vi "daq_run.vi"() -> ()   [LabVIEW 2011]
uses:
  <vilib>/DAQmx/read.llb/DAQmx Read (Analog 1D Wfm NChan NSamp).vi
  <vilib>/DAQmx/miscellaneous.llb/DAQmx Fill In Error Info.vi
  C:/Program Files (x86)/National Instruments/LabVIEW 2011/resource/objmgr/daqmx.rc
  <vilib>/Analysis/NI_AALBase.lvlib
panel:
  in  "Tab Control":T1(tab)=enum."Start DAQ and Nulling"
  in  "X-factor":dbl[](array[numeric])=[22.48, 0.9]
  in  "Strain Offset Nulling":bool
  in  "Shunting Calibration?":bool caption="Shunting Calibration? (DO after nulling)"
  in  "Offset reading":bool
  out "Null_offset":dbl[](array[numeric])=[0.01475870289296967, -9.76222778184623e-05]
  out "Gain adjust":dbl[](array[numeric])
  in  "Sample to read each time":i32=20
  in  "Measure actual excitation?":bool
  in  "Shunt Resistance":dbl=100000.0 format="%0.2f"
  in  "Shunt Location":enum32{"R1", "R2", "R3", "R4"}(ring)=enum."R3"
  out "VOLTAGE":dbl[][](graph)=[[0.3317756410339582, -8.786005003661606e-05]] caption="Voltage based transducer Reading"
  out "Strain Value":dbl[][](graph) caption="Strain gauge readings"
  out "Voltage":dbl[](array[numeric])=[0.3317756410339582, -8.786005003661606e-05]
  out "Strain":dbl[](array[numeric])
  out "Available data points each channel \n(too big will cause overflow problem)":u32
  in  "Record\nfull data to file":bool
  out "Offset indicator":bool
  out "Available data points each channel \n(too big will cause overflow problem) 2":u32
  in  "names in 2":string[](array[string])
  in  "gain":dbl format="%0.2f"
  in  "Boolean":bool
  in  "names in":string[](array[string])
  in  "index":i32
  in  "Path":path
  # "USER's INSTRUCTIONS\n\n1. This Version of of DAQ was developed based on the following hardware combination. Use any of the hardware outside of the following list need further verification \n--- PCI-MIO-16E-4\n--- NI-SCXI-1000/1001\n--- NI-SCXI-1520\n--- NI-SCXI-1314\n\n2. General Steps to use this DAQ software\nStep 1: Click to run the main program (DAQ has not been started yet)\nStep 2: Go over the 'Voltage Channel Initialize' and 'Strain Channel initialize' tab to make  \n             the measurement settings.  click the 'Do parsameter initialize' at least once to set \n             total channels need for voltage and strain, and then change to the right setting.\nStep 3: After all settings, go 'Start DAQ and Nulling' tab and select the sampling rate. After \n             that switch on the 'Start DAQ' button (Will show as green). It is only valid once,if \n             someting goes wrong, abort the execution and run the program again. You can \n             directly approach to Step 3 if all settings in step 2 are correct.\nStep 4: If there is at least one strain gauge channel, hit 'strain offset nulling'  and wait until \n             the gren light turned off. Then shnut calibrate the gauges if need. Finally, turn on \n              'offset reading' to zero the voltage based results. (The ligh will and should be \n             lighted during the following steps.\nStep 5:  Go to tab 'Data monitoring and recording' to see the real time collected data, The \n              voltaged based transducer readings and the strain gauge readings are shown in  \n              separate plots. The Volatge based transducer show the factored value in specific \n              units and the strain shown in microstrain.  \nStep 6: If the data is correctly read. Do the following to initialize the testing:\n             1) Zero the loading machine transducer (UTM,MTS)\n             2) repeat Step 4,5 to rezero all readings in DAQ.\n             3) Click 'Record full data to file' button under 'Data Monitoring and recording' tab\n             4) Run the testing procedure built in UTM or MTS.\nStep 7: Use 'Custom_plot' tab to plot any x versus y plot during the test. \n             USe reset graph to replot, ( the replot will NOT affect the data recording)\nStep 8: turn off the program using 'Start DAQ' button. The data recording to file will switch \n              off simutaneously.\nStep 9: Rename the recorded file, the original name will be this vi file name with 'lvm' \n             extension, can be open with MS.excel\n3. hardware settings\n     Correct Hardware connections are impotant to successul DAQ work. And the setting need to be corresponding to the software settings. The following are common settings:\n\n            1) Pure Voltage (TUM,MTS load and disp export)  :  Half bridge with excitation lead \n                                      unwire)\n            2) Potential meters :  Half bridge with exciation lead wired\n            \n            3) Strain gauge: (Quarter bridge type II is the most commonly used)\n                  See cover of SCXI-1314 for lead connection type for different gauges\nIt is always a good practice to open cover and check the wiring if not sure about that\n\nCOPY this file with 'myshunt.dll' if want to work at other directory\n\n\n4 For more information, check the documents."
  # "Version 2010.5.1\nWrote and compiled by Jun\nemail:xiajun19800812@hotmail.com"
  # "reading scale"
  # "Predefined y=x custom scale"
  # "user factors"
  # "Name and pyhsical channel"
  # "Exciations"
  # "Strain Gauge information"
  # "Reading range"
  # "Channel name and physical address"
  # "bridge settings"
  # "Sampling Frequency, recorded data time spacing is [1/(n2/n1)] second"
  # "Start DAQ"
  # "n1, the number of data to be averaged"
  # "n2, The number collect by DAQ per second"
  # "Strain Channel nulling and shunt calibration"
  # "All Channel numerical offset to zero"
  # "Shunt Calibration information"
  # "Record to file in progress\nWarning:Existing file will be overwrite, change the name below"
  # "Numerical offset in progress"
  # "Peak Valley Detection"
  # "Step 1: Set initial cycle number"
  # "Step 2: Setup cycle detecting alogrithm"
  # "Data Recording"
  # "Step 3: Setup data file recording"
  # "Recording every N cycles for M continuous cycles\nRecord First I cycles completely"
  # "Step 4: Specimen name and start fatigue DAQ"
  # "Remember to create this folder first"
  # "Fatigue recorded file loader"
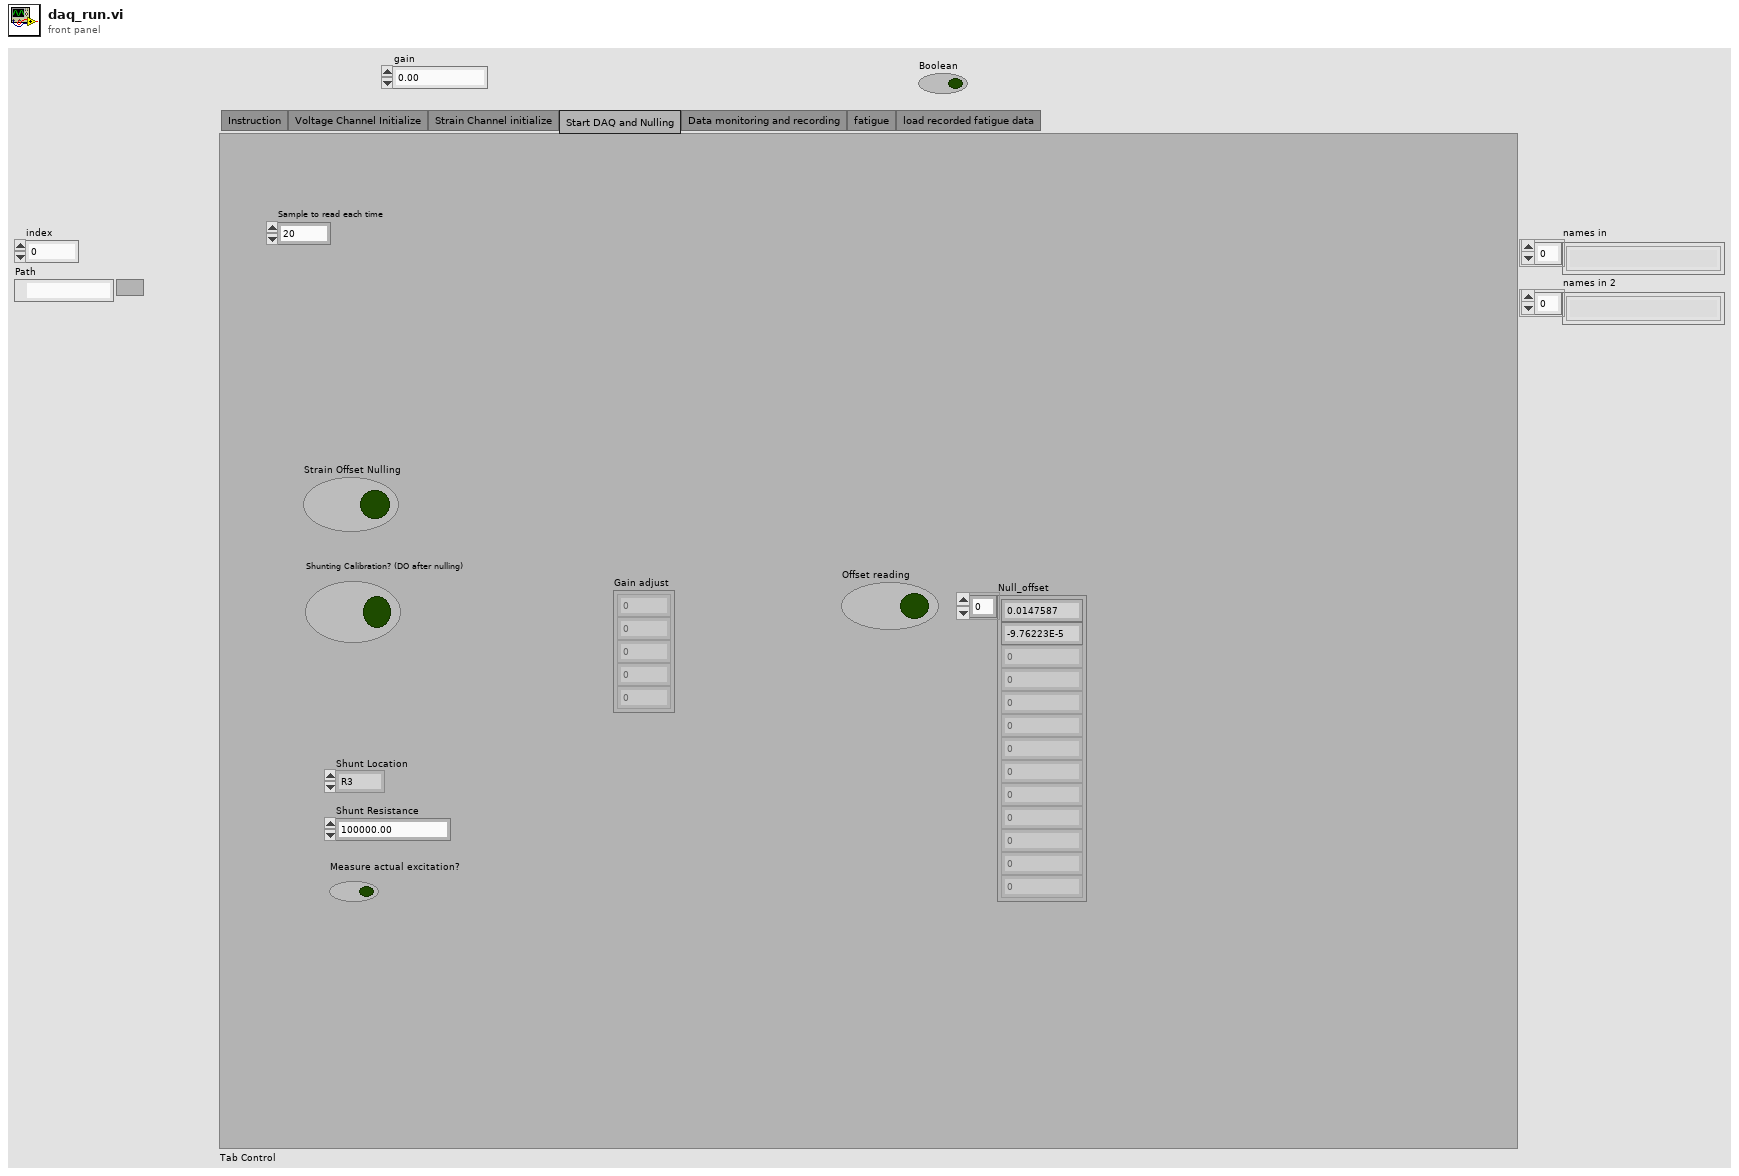
[diagram p1: front panel]
types:
  T1 = enum32{"Instruction", "Voltage Channel Initialize", "Strain Channel initialize", "Start DAQ and Nulling", "Data monitoring and recording", "fatigue", "load recorded fatigue data"}
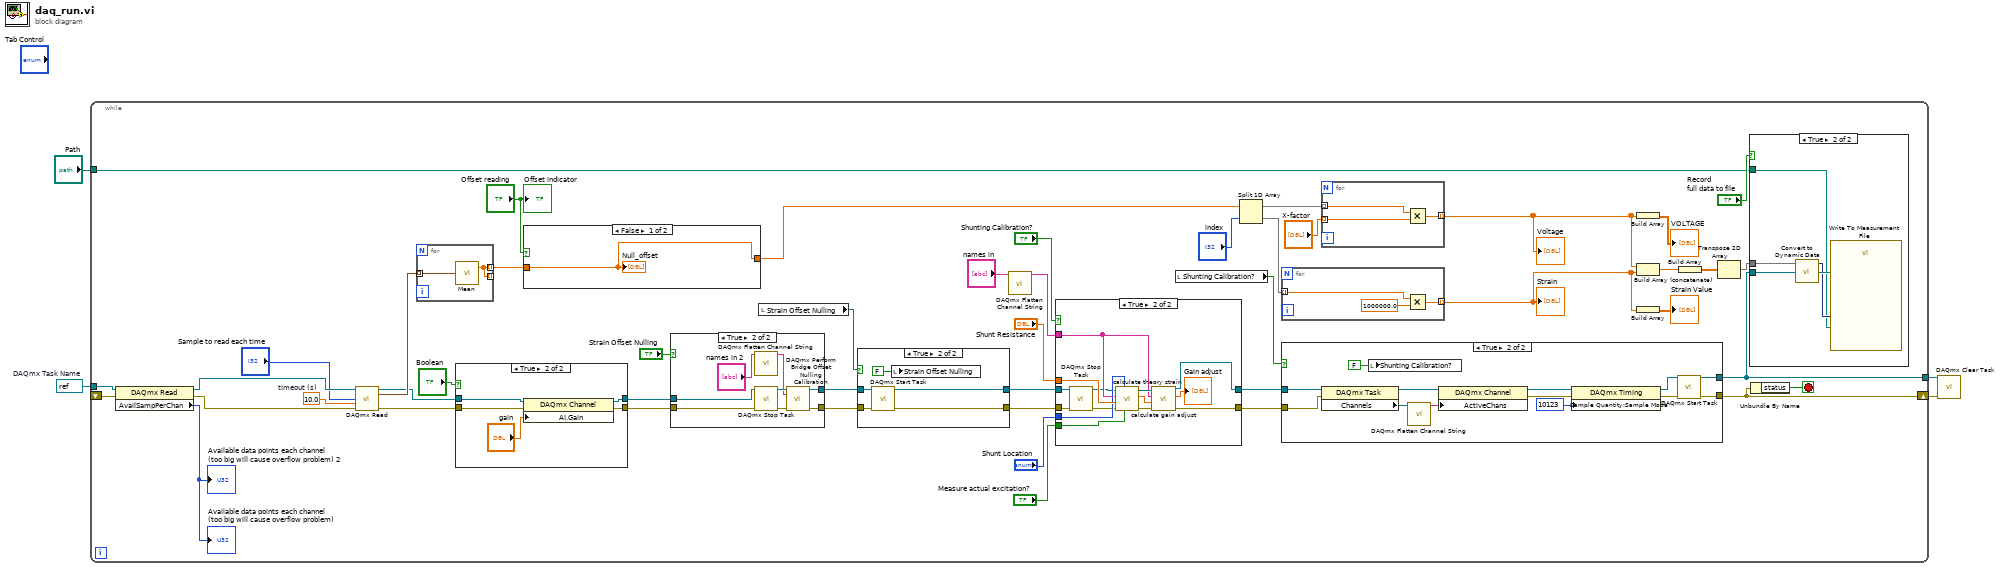
[diagram p0: block diagram]
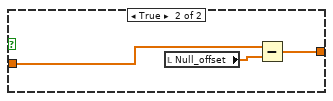
[diagram p3: hidden frame]
diagram:
  w2 = refnum<k21> refnum  # DAQmx Task Name
  n1 = while {
    shift-right: [w32] -> w4
    shift-left: _ -> [w27]
    tunnel: [w28] -> w3
    tunnel: "Path" -> [w31]
    tunnel: w2 -> [w8]
    stop <- w7 stop-if-true
    w20 = 10.0  # timeout (s)
    n2 = property class="DAQmx Read"(reference=w8, error in=w27) -> (reference out=w26:refnum<k21>, error out=w25:errorcluster, "AvailSampPerChan"=→"Available data points each channel \n(too big will cause overflow problem)" →"Available data points each channel \n(too big will cause overflow problem) 2":u32)
    n3 = call-poly <vilib>:"DAQmx Read.vi"("task/channels in"=w26, "number of samples per channel"="Sample to read each time", "timeout"=w20, "error in"=w25) -> ("task out"=w12:refnum<k21>, "data"=w15:waveform(dbl)[], "error out"=w13:errorcluster)  [unwired: 9 out]
    n4 = for {
      tunnel: w15 -> [w59] mode=indexing
      tunnel: [w60] -> _ mode=indexing
      tunnel: [w60] -> w21 mode=indexing
      n5 = call <vilib>:"Mean.vi"("X"=w59) -> ("mean"=w60:dbl)  [unwired: 1 out]
    }
    n6 = case shown="True" "Boolean" {
      tunnel: [w52 w54] -> w9
      tunnel: w13 -> [w52 w57]
      tunnel: w12 -> [w53 w56]
      tunnel: [w53 w55] -> w11
      frame False {
      }
      frame True {
        n7 = property class="DAQmx Channel"(reference=w56, error in=w57, "AI.Gain"="gain") -> (reference out=w55:refnum<k21>, error out=w54:errorcluster)
      }
    }
    n8 = case shown="False" "Offset reading" {
      tunnel: w21 -> [w61 w64]
      tunnel: [w61 w62] -> w23
      frame False {
        "Null_offset" <- w61
      }
      frame True {
        n9 = local read "Null_offset"() -> (w63:dbl[])
        n10 = Subtract(x=w64, y=w63) -> (x-y=w62:dbl[])
      }
    }
    n11 = case shown="True" "Strain Offset Nulling" {
      tunnel: w11 -> [w114 w121]
      tunnel: [w114 w122] -> w49
      tunnel: [w113 w117] -> w10
      tunnel: w9 -> [w113 w116]
      frame False {
      }
      frame True {
        n12 = call <vilib>:"DAQmx Flatten Channel String.vi"("names in"="names in 2") -> ("names out"=w118:string)  [unwired: 1 in, 13 out]
        n13 = call <vilib>:"DAQmx Stop Task.vi"("task/channels in"=w121, "error in"=w116) -> ("task out"=w120:refnum<k21>, "error out"=w119:errorcluster)  [unwired: 12 out]
        n14 = call <vilib>:"DAQmx Perform Bridge Offset Nulling Calibration.vi"("task/channels in"=w120, "channels"=w118, "error in"=w119) -> ("task out"=w122:refnum<k21>, "error out"=w117:errorcluster)  [unwired: 1 in, 10 out]
      }
    }
    n15 = local read "Strain Offset Nulling"() -> (w50:bool)
    n16 = case shown="True" w50 {
      tunnel: w49 -> [w107 w111]
      tunnel: [w107 w110] -> w37
      tunnel: [w106 w108] -> w36
      tunnel: w10 -> [w106 w109]
      frame False {
      }
      frame True {
        n17 = call <vilib>:"DAQmx Start Task.vi"("task/channels in"=w111, "error in"=w109) -> ("task out"=w110:refnum<k21>, "error out"=w108:errorcluster)  [unwired: 12 out]
        n18 = local write "Strain Offset Nulling"(FALSE) -> ()
      }
    }
    n19 = call <vilib>:"DAQmx Flatten Channel String.vi"("names in"="names in") -> ("names out"=w39:string)  [unwired: 1 in, 13 out]
    n20 = case shown="True" "Shunting Calibration?" {
      tunnel: [w80 w88] -> w35
      tunnel: [w81 w87] -> w34
      tunnel: w36 -> [w81 w84]
      tunnel: w39 -> [_ w89]
      tunnel: "Shunt Resistance" -> [_ w95]
      tunnel: "Shunt Location" -> [_ w94]
      tunnel: "Measure actual excitation?" -> [_ w93]
      tunnel: w37 -> [w80 w85]
      frame False {
      }
      frame True {
        n21 = call <vilib>:"DAQmx Stop Task.vi"("task/channels in"=w85, "error in"=w84) -> ("task out"=w83:refnum<k21>, "error out"=w82:errorcluster)  [unwired: 12 out]
        n22 = call "calculate theory strain.vi"("Measure actual excitation?"=w93, "Shunt Location"=w94, "error in"=w82, "Shunt Resistance"=w95, "Channels"=w89, "task in"=w83) -> ("error out"=w91:errorcluster, "Theory strain value"=w90:dbl[], "task out"=w92:refnum<k21>)  [unwired: 1 in, 2 out]
        n23 = call "calculate gain adjust.vi"("error in"=w91, "Theoretical Strains"=w90, "Channels"=w89, "task in"=w92) -> ("error out"=w87:errorcluster, "Gain adjust"=→"Gain adjust":dbl[], "task out"=w88:refnum<k21>)  [unwired: 5 out]
      }
    }
    n24 = local read "Shunting Calibration?"() -> (w33:bool)
    n25 = Split 1D Array(array=w23, index="index") -> (first subarray=w46:dbl[], second subarray=w45:dbl[])
    n26 = for {
      tunnel: w45 -> [w98] mode=indexing
      tunnel: [w96] -> w43 mode=indexing
      n27 = Multiply(x=w98, y=1000000.0) -> (x*y=w96:dbl)
    }
    "Strain" <- w43
    n28 = case shown="True" w33 {
      tunnel: w35 -> [w66 w74]
      tunnel: [w66 w72] -> w28
      tunnel: [w65 w78] -> w32
      tunnel: w34 -> [w65 w73]
      frame False {
      }
      frame True {
        n29 = property class="DAQmx Task"(reference=w74, error in=w73) -> (reference out=w76:refnum<k21>, "Channels"=w77:refnum<k21>[])  [unwired: 1 out]
        n30 = local write "Shunting Calibration?"(FALSE) -> ()
        n31 = call <vilib>:"DAQmx Flatten Channel String.vi"("names in"=w77) -> ("names out"=w75:string)  [unwired: 1 in, 13 out]
        n32 = property class="DAQmx Channel"(reference=w76, "ActiveChans"=w75) -> (reference out=w69:refnum<k21>, error out=w68:errorcluster)  [unwired: 1 in]
        n33 = property class="DAQmx Timing"(reference=w69, error in=w68, "Sample Quantity:Sample Mode"=10123) -> (reference out=w71:refnum<k21>, error out=w70:errorcluster)
        n34 = call <vilib>:"DAQmx Start Task.vi"("task/channels in"=w71, "error in"=w70) -> ("task out"=w72:refnum<k21>, "error out"=w78:errorcluster)  [unwired: 12 out]
      }
    }
    n35 = for {
      tunnel: "X-factor" -> [w100] mode=indexing
      tunnel: w46 -> [w101] mode=indexing
      tunnel: [w99] -> w44 mode=indexing
      n36 = Multiply(x=w101, y=w100) -> (x*y=w99:dbl)
    }
    "Voltage" <- w44
    n37 = Build Array(w44) -> (→"VOLTAGE":dbl[][])
    n38 = Build Array (concatenate)(w44, w43) -> (w18:dbl[])
    n39 = Build Array(w43) -> (→"Strain Value":dbl[][])
    n40 = Build Array(w18) -> (w19:dbl[][])
    n41 = Transpose 2D Array(2D array=w19) -> (transposed array=w17:dbl[][])
    n42 = case shown="True" "Record\nfull data to file" {
      tunnel: w31 -> [_ w102]
      tunnel: w17 -> [_ w104]
      tunnel: w28 -> [_ w105]
      frame False {
      }
      frame True {
        n43 = call "Convert to Dynamic Data"("2D Array"=w104) -> ("Dynamic Data Type"=w103:dynamicdata)  [unwired: 3 out]
        n44 = call "Write To Measurement File"("Signals"=w103, "File Name"=w102, "DAQmx Task"=w105) -> ()  [unwired: 4 in, 13 out]
      }
    }
    n45 = Unbundle By Name(w32) -> ("status"=w7:bool)
    "Offset indicator" <- "Offset reading"
  }
  n46 = call <vilib>:"DAQmx Clear Task.vi"("task in"=w3, "error in"=w4) -> ()  [unwired: 14 out]
